vi "N4.vi"() -> ()   [LabVIEW 2020]
uses:
  <vilib>/numeric/Random Number (Range) U64.vi
  <vilib>/numeric/sub_Random U32.vi
panel:
  out "Array":u64[](array[numeric])
  out "Index":i32[](array[numeric])
  out "MAX":u64[](array[numeric])
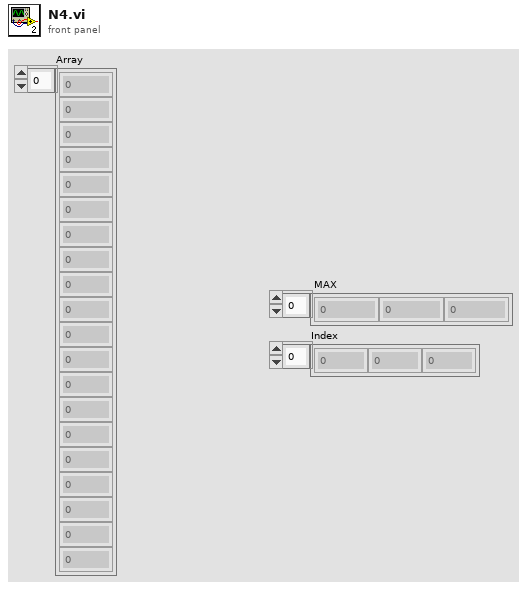
[diagram p1: front panel]
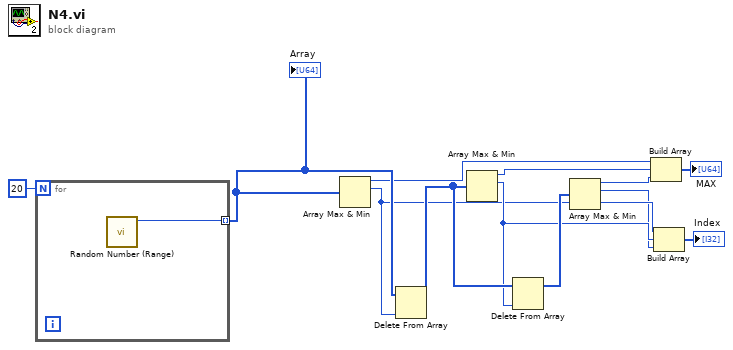
[diagram p0: block diagram]
diagram:
  n1 = for {
    N: 20 -> [_]
    tunnel: [w13] -> w12 mode=indexing
    n2 = call-poly <vilib>:"Random Number (Range).vi"() -> ("number"=w13:u64)  [unwired: 11 in]
  }
  "Array" <- w12
  n3 = Array Max & Min(array=w12) -> (max value=w11:u64, max index (indices)=w4:i32)  [unwired: 2 out]
  n4 = Delete From Array(array=w12, index=w4) -> (array with subset deleted=w8:u64[])  [unwired: 1 in, 1 out]
  n5 = Array Max & Min(array=w8) -> (max value=w10:u64, max index (indices)=w5:i32)  [unwired: 2 out]
  n6 = Delete From Array(array=w8, index=w5) -> (array with subset deleted=w9:u64[])  [unwired: 1 in, 1 out]
  n7 = Array Max & Min(array=w9) -> (max value=w7:u64, max index (indices)=w3:i32)  [unwired: 2 out]
  n8 = Build Array(w11, w10, w7) -> (→"MAX":u64[])
  n9 = Build Array(w4, w5, w3) -> (→"Index":i32[])
